vi "Configure9214.vi"(7 "Channel Number":i32, 8 "error in (no error)":errorcluster, 10 "Properties":T1[](array[typedef]), 11 "IO Ref":refnum<k21>) -> (0 "error out":errorcluster, 3 "IO Ref out":refnum<k21>)   [LabVIEW 2017, in "ScanEngine.lvlib"]
uses:
  <vilib>/addons/InsightCM/Devices/Shared/Common/ScanEngine/ScanEngine.lvlib
  <vilib>/addons/InsightCM/MessageBus/Base/controls/KeyValuePair.ctl
  <resource>/objmgr/cRIO.rc
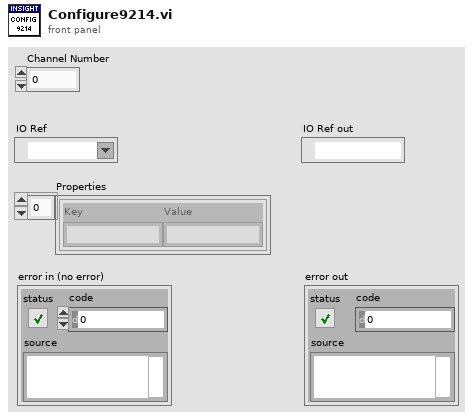
[diagram p1: front panel]
types:
  T1 = typedef "KeyValuePair.ctl" = cluster{"Key":string, "Value":string}
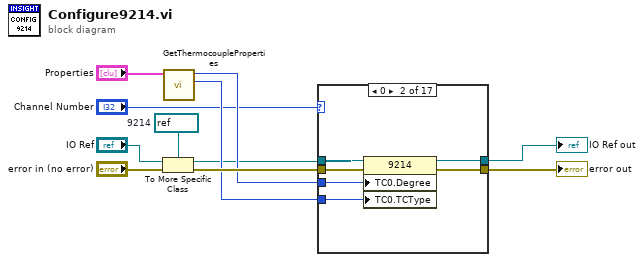
[diagram p0: block diagram]
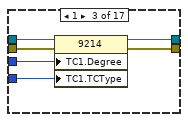
[diagram p3: hidden frame]
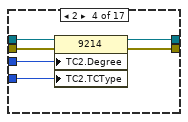
[diagram p4: hidden frame]
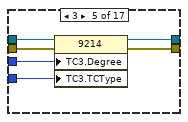
[diagram p5: hidden frame]
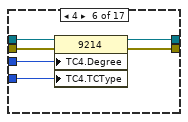
[diagram p6: hidden frame]
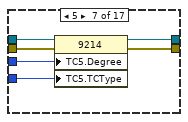
[diagram p7: hidden frame]
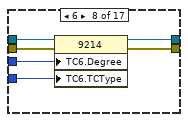
[diagram p8: hidden frame]
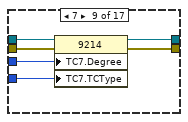
[diagram p9: hidden frame]
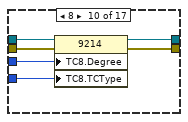
[diagram p10: hidden frame]
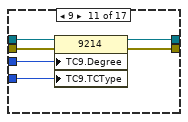
[diagram p11: hidden frame]
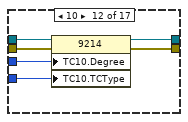
[diagram p12: hidden frame]
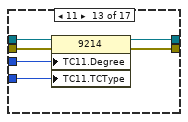
[diagram p13: hidden frame]
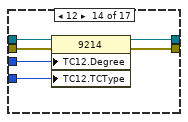
[diagram p14: hidden frame]
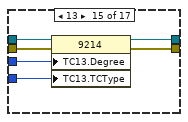
[diagram p15: hidden frame]
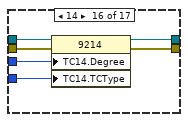
[diagram p16: hidden frame]
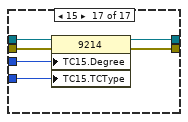
[diagram p17: hidden frame]
diagram:
  w3 = refnum<k21> refnum  # 9214
  n1 = To More Specific Class(target class=w3, reference="IO Ref", error in="error in (no error)") -> (specific class reference=w4:refnum<k21>, error out=w11:errorcluster)
  n2 = call <vilib>:"GetThermocoupleProperties.vi"("Properties"="Properties") -> ("AI Thermocouple type"=w10:u32, "AI degree range"=w9:u32)  [unwired: 9 in]
  n3 = case shown="0" "Channel Number" {
    tunnel: w11 -> [w13 w16 w22 w28 w34 w40 w46 w52 w58 w64 w70 w76 w82 w88 w94 w100 w106]
    tunnel: [w13 w19 w25 w31 w37 w43 w49 w55 w61 w67 w73 w79 w85 w91 w97 w103 w109] -> w6
    tunnel: w9 -> [_ w18 w24 w30 w36 w42 w48 w54 w60 w66 w72 w78 w84 w90 w96 w102 w108]
    tunnel: w10 -> [_ w17 w23 w29 w35 w41 w47 w53 w59 w65 w71 w77 w83 w89 w95 w101 w107]
    tunnel: w4 -> [w12 w15 w21 w27 w32 w39 w45 w51 w57 w63 w69 w75 w81 w87 w93 w99 w105]
    tunnel: [w12 w14 w20 w26 w33 w38 w44 w50 w56 w62 w68 w74 w80 w86 w92 w98 w104] -> w7
    frame -1, Default {
    }
    frame 0 {
      n4 = property class="9214"(reference=w15, error in=w16, "TC0.Degree"=w18, "TC0.TCType"=w17) -> (reference out=w14:refnum<k21>, error out=w19:errorcluster)
    }
    frame 1 {
      n5 = property class="9214"(reference=w21, error in=w22, "TC1.Degree"=w24, "TC1.TCType"=w23) -> (reference out=w20:refnum<k21>, error out=w25:errorcluster)
    }
    frame 2 {
      n6 = property class="9214"(reference=w27, error in=w28, "TC2.Degree"=w30, "TC2.TCType"=w29) -> (reference out=w26:refnum<k21>, error out=w31:errorcluster)
    }
    frame 3 {
      n7 = property class="9214"(reference=w32, error in=w34, "TC3.Degree"=w36, "TC3.TCType"=w35) -> (reference out=w33:refnum<k21>, error out=w37:errorcluster)
    }
    frame 4 {
      n8 = property class="9214"(reference=w39, error in=w40, "TC4.Degree"=w42, "TC4.TCType"=w41) -> (reference out=w38:refnum<k21>, error out=w43:errorcluster)
    }
    frame 5 {
      n9 = property class="9214"(reference=w45, error in=w46, "TC5.Degree"=w48, "TC5.TCType"=w47) -> (reference out=w44:refnum<k21>, error out=w49:errorcluster)
    }
    frame 6 {
      n10 = property class="9214"(reference=w51, error in=w52, "TC6.Degree"=w54, "TC6.TCType"=w53) -> (reference out=w50:refnum<k21>, error out=w55:errorcluster)
    }
    frame 7 {
      n11 = property class="9214"(reference=w57, error in=w58, "TC7.Degree"=w60, "TC7.TCType"=w59) -> (reference out=w56:refnum<k21>, error out=w61:errorcluster)
    }
    frame 8 {
      n12 = property class="9214"(reference=w63, error in=w64, "TC8.Degree"=w66, "TC8.TCType"=w65) -> (reference out=w62:refnum<k21>, error out=w67:errorcluster)
    }
    frame 9 {
      n13 = property class="9214"(reference=w69, error in=w70, "TC9.Degree"=w72, "TC9.TCType"=w71) -> (reference out=w68:refnum<k21>, error out=w73:errorcluster)
    }
    frame 10 {
      n14 = property class="9214"(reference=w75, error in=w76, "TC10.Degree"=w78, "TC10.TCType"=w77) -> (reference out=w74:refnum<k21>, error out=w79:errorcluster)
    }
    frame 11 {
      n15 = property class="9214"(reference=w81, error in=w82, "TC11.Degree"=w84, "TC11.TCType"=w83) -> (reference out=w80:refnum<k21>, error out=w85:errorcluster)
    }
    frame 12 {
      n16 = property class="9214"(reference=w87, error in=w88, "TC12.Degree"=w90, "TC12.TCType"=w89) -> (reference out=w86:refnum<k21>, error out=w91:errorcluster)
    }
    frame 13 {
      n17 = property class="9214"(reference=w93, error in=w94, "TC13.Degree"=w96, "TC13.TCType"=w95) -> (reference out=w92:refnum<k21>, error out=w97:errorcluster)
    }
    frame 14 {
      n18 = property class="9214"(reference=w99, error in=w100, "TC14.Degree"=w102, "TC14.TCType"=w101) -> (reference out=w98:refnum<k21>, error out=w103:errorcluster)
    }
    frame 15 {
      n19 = property class="9214"(reference=w105, error in=w106, "TC15.Degree"=w108, "TC15.TCType"=w107) -> (reference out=w104:refnum<k21>, error out=w109:errorcluster)
    }
  }
  "IO Ref out" <- w7
  "error out" <- w6
